vi "WMI_SetDefaultPrinters.vi"(8 "error in (no error)":errorcluster, 11 "PrinterName":string) -> (0 "error out":errorcluster, 2 "Found?":bool)   [LabVIEW 2021]
doc: "This VI sets the default printer specified by name."
uses:
  System.Management
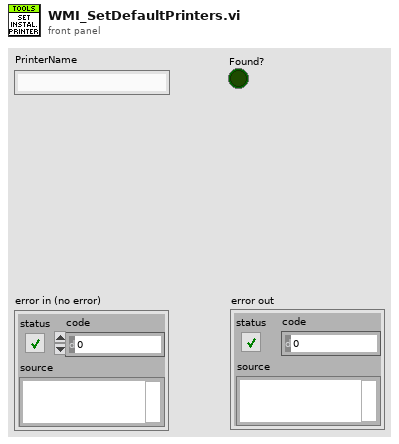
[diagram p1: front panel]
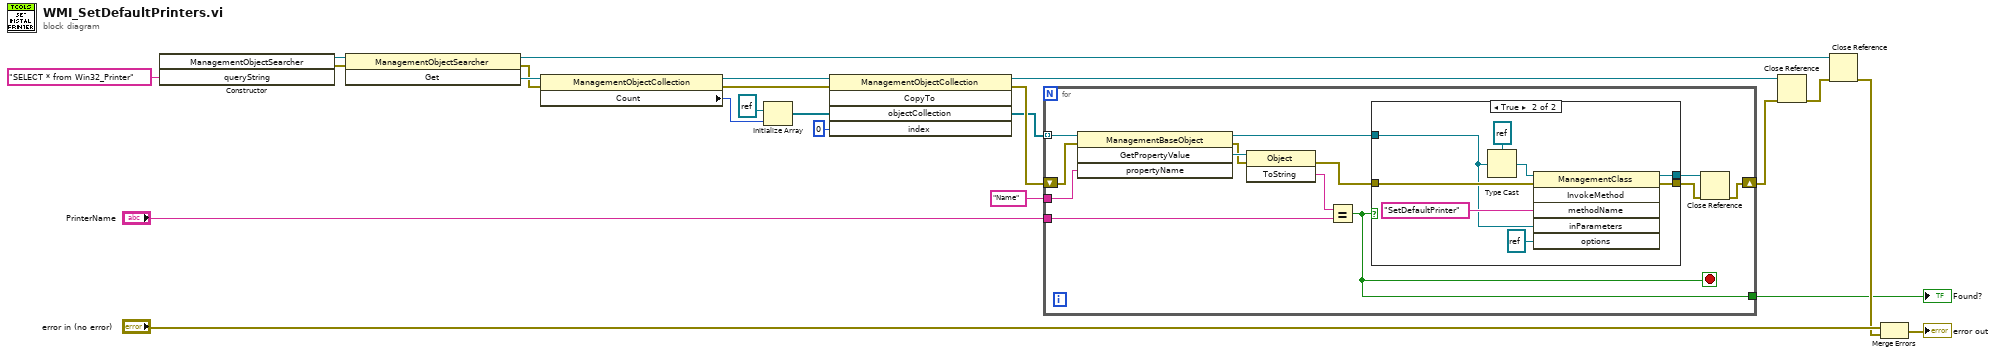
[diagram p0: block diagram]
diagram:
  n1 = constructor class="ManagementObjectSearcher"("queryString"="SELECT * from Win32_Printer" ("scope")) -> (reference out=w22:refnum<k24>, error out=w21:errorcluster)  [unwired: 3 in, 2 out]
  n2 = invoke class="ManagementObjectSearcher" method="Get"(reference=w22, error in=w21) -> (reference out=w20:refnum<k24>, error out=w8:errorcluster, "Get"=w16:refnum<k24>)  [unwired: 1 in]
  n3 = property class="ManagementObjectCollection"(reference=w16, error in=w8) -> (reference out=w11:refnum<k24>, error out=w10:errorcluster, "Count"=w14:i32)
  n4 = Initialize Array(refnum<k24> refnum, w14) -> (w12:refnum<k24>[])
  n5 = invoke class="ManagementObjectCollection" method="CopyTo"(reference=w11, error in=w10, "objectCollection"=w12, "index"=0) -> (reference out=w3:refnum<k24>, error out=w9:errorcluster, "objectCollection"=w7:refnum<k24>[])  [unwired: 1 in, 2 out]
  n6 = for {
    shift-right: [w35] -> w2
    shift-left: w9 -> [w33]
    tunnel: w7 -> [w31] mode=indexing
    tunnel: "Name" ("propertyName") -> [w30]
    tunnel: "PrinterName" -> [w25]
    tunnel: [w24] -> w4
    stop <- w24 stop-if-true
    n7 = invoke class="ManagementBaseObject" method="GetPropertyValue"(reference=w31, error in=w33, "propertyName"=w30) -> (reference out=w32:refnum<k24>, error out=w28:errorcluster, "GetPropertyValue"=w29:refnum<k24>)  [unwired: 1 in, 1 out]
    n8 = invoke class="Object" method="ToString"(reference=w29, error in=w28) -> (error out=w27:errorcluster, "ToString"=w26:string)  [unwired: 1 in, 1 out]
    n9 = Equal?(x=w26, y=w25) -> (x = y?=w24:bool)
    n10 = case shown="True" w24 {
      tunnel: w27 -> [w37 w43]
      tunnel: w32 -> [w38 w41]
      tunnel: [w37 w40] -> w36
      tunnel: [w38 w39] -> w34
      frame False {
      }
      frame True {
        n11 = Type Cast(type=refnum<k24> refnum ("reference"), x=w41) -> (*(type *) &x=w45:refnum<k24>)
        n12 = invoke class="ManagementClass" method="InvokeMethod"(reference=w45, error in=w43, "methodName"="SetDefaultPrinter", "inParameters"=w41, "options"=refnum<k24> refnum) -> (reference out=w39:refnum<k24>, error out=w40:errorcluster)  [unwired: 1 in, 4 out]
      }
    }
    n13 = Close Reference(reference=w34, error in (no error)=w36) -> (error out=w35:errorcluster)
  }
  "Found?" <- w4
  n14 = Close Reference(reference=w3, error in (no error)=w2) -> (error out=w1:errorcluster)
  n15 = Close Reference(reference=w20, error in (no error)=w1) -> (error out=w17:errorcluster)
  n16 = Merge Errors("error in (no error)", w17) -> (→"error out":errorcluster)
